vi "Scale Channel.vi"(8 "error in (no error)":errorcluster, 9 "Instance":string, 10 "Value In":dbl, 11 "Polynomial in":refnum<class "Polynomial.lvclass">) -> (0 "error out":errorcluster, 2 "Value Out":dbl, 3 "Polynomial out":refnum<class "Polynomial.lvclass">)   [LabVIEW 2018, in "Polynomial.lvclass"]
doc: "Polynomial.lvclass:Scale Channel.vi\n\nThis VI scales a single Channel using a Polynomial scaling.\n\nInstrument Communication Module Version 1.0\nNovember, 2017 Original Code Consulting David Thomson\n www.originalcode.com David Thomson"
uses:
  Polynomial.lvclass
  Polynomial.lvclass/Polynomial.ctl
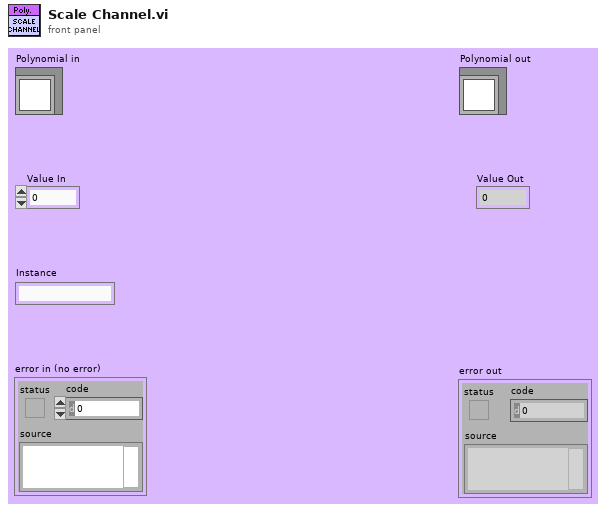
[diagram p1: front panel]
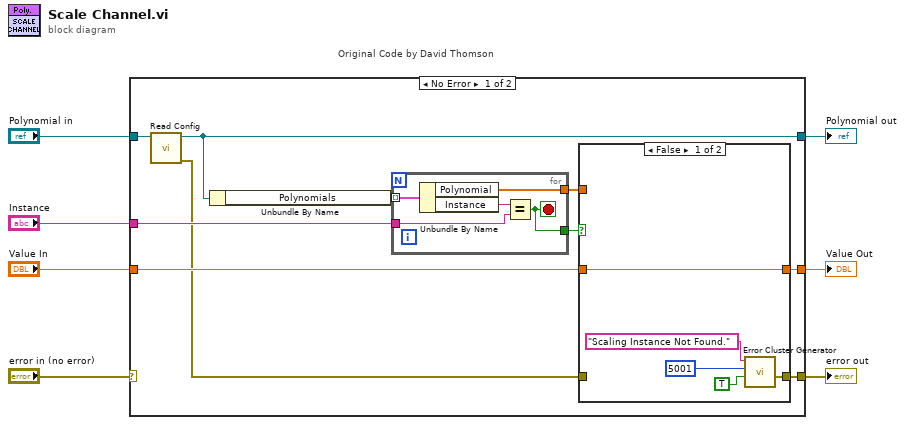
[diagram p0: block diagram]
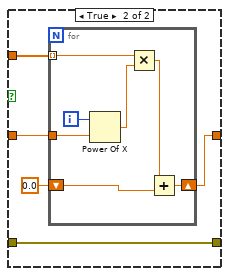
[diagram p2: hidden frame]
diagram:
  n1 = case "Original Code by David Thomson" shown="No Error" "error in (no error)" {
    selector: "error in (no error)" -> [_ w42]
    tunnel: [w14 w42] -> w6
    tunnel: [w9 w41] -> w4
    tunnel: "Polynomial in" -> [w10 w41]
    tunnel: "Instance" -> [w17 _]
    tunnel: "Value In" -> [w12 w40]
    tunnel: [w13 w40] -> w1
    frame No Error {
      n2 = call-dynamic "Read Config.vi"("Polynomial in"=w10) -> ("error out"=w8:errorcluster, "Polynomial out"=w9:refnum<class "Polynomial.lvclass">)  [unwired: 9 in]
      n3 = Unbundle By Name(w9) -> ("Polynomials"=w16:cluster{"Instance":string, "Polynomial":dbl[]}[])
      n4 = for {
        tunnel: w17 -> [w37]
        tunnel: w16 -> [w39] mode=indexing
        tunnel: [w36] -> w15
        tunnel: [w35] -> w11
        stop <- w36 stop-if-true
        n5 = Unbundle By Name(w39) -> ("Polynomial"=w35:dbl[], "Instance"=w38:string)
        n6 = Equal?(x=w38, y=w37) -> (x = y?=w36:bool)
      }
      n7 = case shown="False" w15 {
        tunnel: w8 -> [_ w27]
        tunnel: [w21 w27] -> w14
        tunnel: [w22 w25] -> w13
        tunnel: w12 -> [w22 w23]
        tunnel: w11 -> [_ w24]
        frame False {
          n8 = call "Error Cluster Generator.vi"("Error (T)"=TRUE, "code"=5001, "Additional message"="Scaling Instance Not Found.") -> ("error out"=w21:errorcluster)  [unwired: 3 in, 1 out]
        }
        frame True {
          n9 = for {
            shift-right: [w34] -> w25
            shift-left: 0.0 ("Value In") -> [w33]
            tunnel: w24 -> [w32] mode=indexing
            tunnel: w23 -> [w29]
            i -> [w28]
            n10 = Power Of X(1:w29, 2:w28) -> (0:w30:dbl)
            n11 = Multiply(x=w32, y=w30) -> (x*y=w31:dbl)
            n12 = Add(x=w31, y=w33) -> (x+y=w34:dbl)
          }
        }
      }
    }
    frame Error {
    }
  }
  "error out" <- w6
  "Polynomial out" <- w4
  "Value Out" <- w1
